vi "Initiate.vi"(8 "error in (no error)":errorcluster, 11 "Tektronix MSO5 in":refnum<class "Tektronix MSO5.lvclass">) -> (0 "error out":errorcluster, 3 "Tektronix MSO5 out":refnum<class "Tektronix MSO5.lvclass">)   [LabVIEW 2025, in "Scope.lvlib" / "Tektronix MSO5.lvclass"]
uses:
  Tektronix MSO5.lvclass
  Tektronix MSO5.lvclass/Tektronix MSO5.ctl
  <instrlib>/Tektronix MSO5X Series/Tektronix MSO5X Series.lvlib
  Scope Instrument/Scope Instrument.lvclass
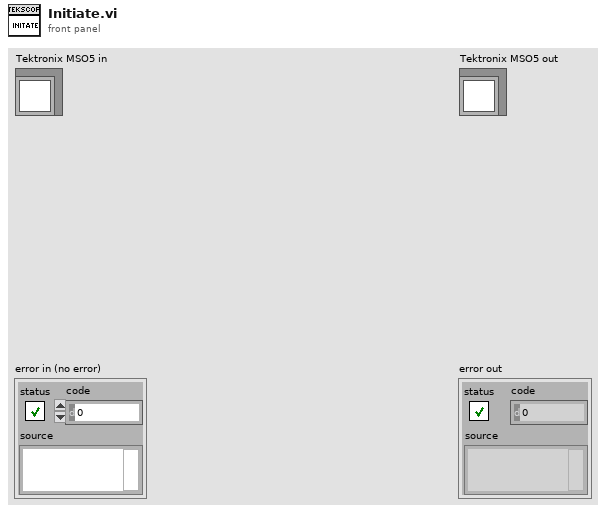
[diagram p1: front panel]
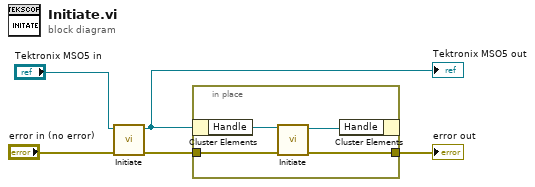
[diagram p0: block diagram]
diagram:
  n1 = call-parent <instrlib>:"Initiate.vi"("error in (no error)"="error in (no error)", "Scope Instrument in"="Tektronix MSO5 in") -> ("error out"=w2:errorcluster, "Scope Instrument out"=w3:refnum<class "Tektronix MSO5.lvclass">)  [unwired: 8 in]
  "Tektronix MSO5 out" <- w3
  n2 = in-place {
    in-place-border: w2 -> [w9]
    in-place-border: [w8] -> w1
    n3 = in-place-cluster #1(w3) -> ("Handle"=w7:refnum<visa-resource-name>)
    n4 = call <instrlib>:"Initiate.vi"("error in (no error)"=w9, "VISA resource name"=w7) -> ("error out"=w8:errorcluster, "VISA resource name out"=w6:refnum<visa-resource-name>)  [unwired: 8 in]
    n5 = in-place-cluster #1("Handle"=w6) -> ()  [unwired: 1 out]
  }
  "error out" <- w1
